vi "Read position mMc.vi"(1 "Port":T1={"P type"=0, "reference"="", " Terminator "="\r\n", "Timeout"=300} {"Timeout" step=10; "P type" items=["none", "RS-232C"]}, 3 "error in (no error)":errorcluster, 5 "Controller #":string) -> (6 "Cnt pos":dbl, 7 "Enc pos":dbl, 9 "error out":errorcluster)   [LabVIEW 2020]
panel:
  # "Read position"
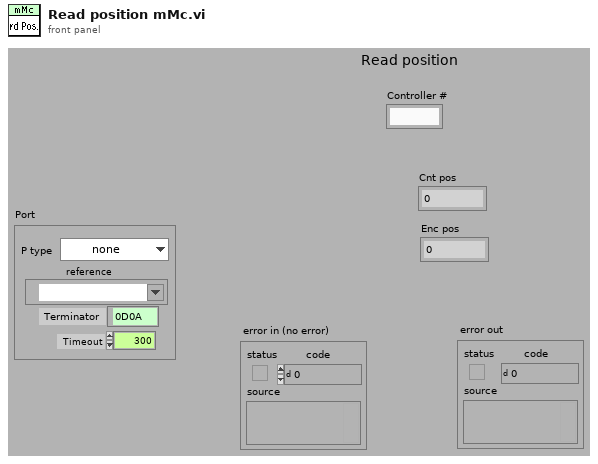
[diagram p1: front panel]
types:
  T1 = cluster{"P type":u16, "reference":refnum<visa-resource-name>, " Terminator ":string, "Timeout":i32}
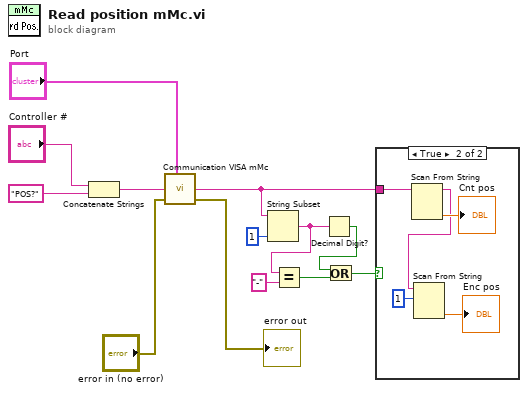
[diagram p0: block diagram]
diagram:
  n1 = Concatenate Strings("Controller #", "POS?") -> (w9:string)
  n2 = call "Communication VISA mMc.vi"("Port"="Port", "Command"=w9, "error in (no error)"="error in (no error)") -> ("Return"=w6:string, "error out"=→"error out":errorcluster)  [unwired: 3 in, 2 out]
  n3 = String Subset(string=w6, length (rest)=1 ("length (rest)")) -> (substring=w5:string)  [unwired: 1 in]
  n4 = Equal?(x=w5, y="-") -> (x = y?=w2:bool)
  n5 = Decimal Digit?(1:w5) -> (0:w3:bool)
  n6 = Or(x=w3, y=w2) -> (x .or. y?=w1:bool)
  n7 = case shown="True" w1 {
    tunnel: w6 -> [_ w17]
    frame False {
    }
    frame True {
      n8 = Scan From String(input string=w17) -> (remaining string=w16:string, output 1=→"Cnt pos":dbl)  [unwired: 4 in, 2 out]
      n9 = Scan From String(input string=w16, initial scan location=u32 1) -> (output 1=→"Enc pos":dbl)  [unwired: 3 in, 3 out]
    }
  }
